vi "Execute.vi"(8 "error in (no error)":errorcluster, 11 "Normalize in":refnum<class "Normalize.lvclass">) -> (0 "error out":errorcluster, 2 "Data":dbl[](array[numeric]), 3 "Normalize out":refnum<class "Normalize.lvclass">)   [LabVIEW 2021, in "Normalize.lvclass"]
uses:
  Normalize.lvclass
  Normalize.lvclass/Normalize.ctl
  Decorator/Decorator.lvclass
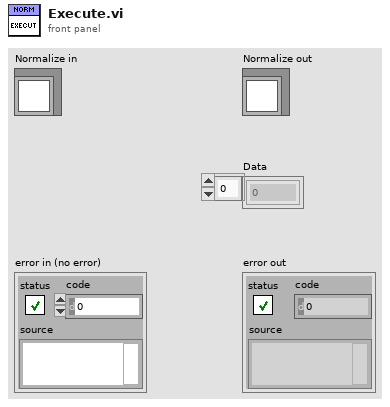
[diagram p1: front panel]
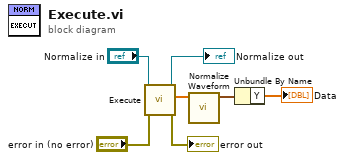
[diagram p0: block diagram]
diagram:
  n1 = call-parent "Execute.vi"("error in (no error)"="error in (no error)", "Decorator in"="Normalize in") -> ("error out"=→"error out":errorcluster, "Data"=w3:dbl[], "Decorator out"=→"Normalize out":refnum<class "Normalize.lvclass">)  [unwired: 7 in]
  n2 = call <vilib>:"Normalize Waveform.vi"("waveform in"=w3) -> ("normalized waveform"=w1:waveform(dbl))  [unwired: 7 in, 3 out]
  n3 = Unbundle By Name(w1) -> ("Y"=→"Data":dbl[])
